vi "Connect to cDAQ.vi"(10 "System":string, 11 "Abort Ref":refnum<vi>) -> (1 "Abort":bool, 2 "Connected?":bool, 3 "System Ref":tag)   [LabVIEW 2023]
uses:
  <resource>/objmgr/daqmx.rc
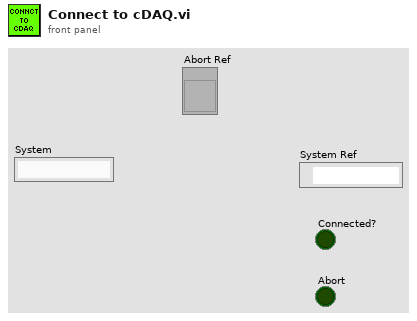
[diagram p1: front panel]
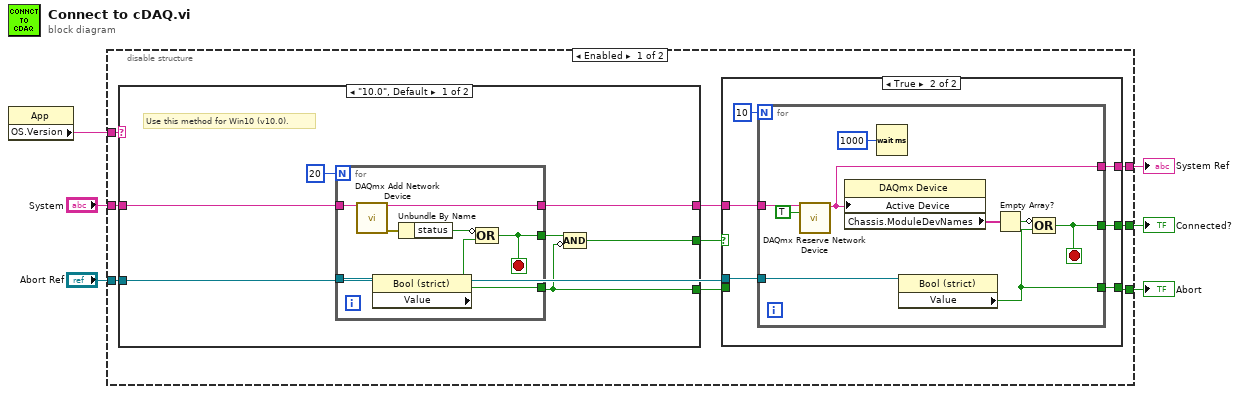
[diagram p0: block diagram]
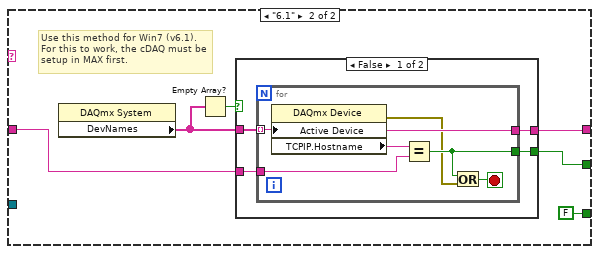
[diagram p2: hidden frame]
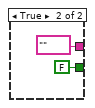
[diagram p3: hidden frame]
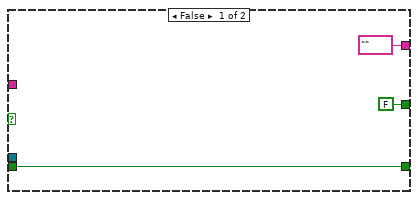
[diagram p4: hidden frame]
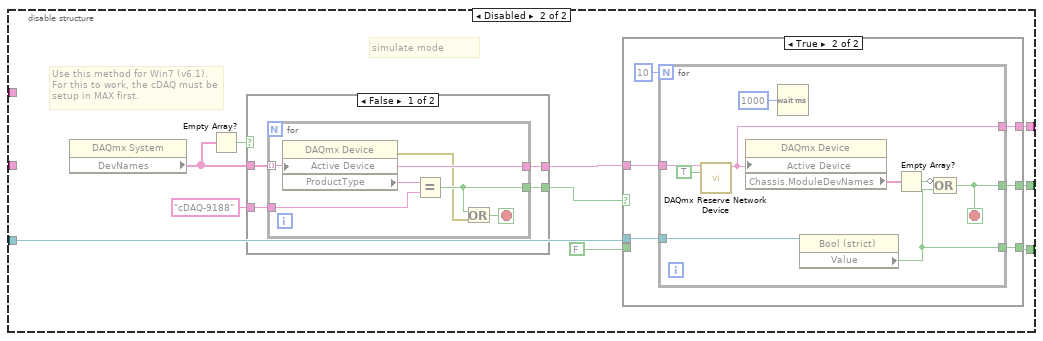
[diagram p5: hidden frame]
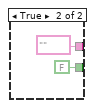
[diagram p6: hidden frame]
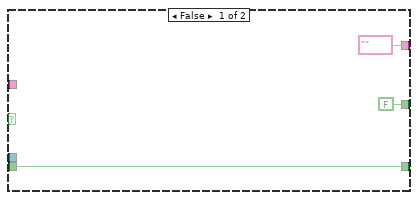
[diagram p7: hidden frame]
diagram:
  n1 = property class="App"() -> ("OS.Version"=w1:string)  [unwired: 2 in, 2 out]
  n2 = disable-structure shown="Enabled" {
    disable-tunnel: "System" -> [w15 _]
    disable-tunnel: [w12 w73] -> w5
    disable-tunnel: [w11 w72] -> w4
    disable-tunnel: [w10 w71] -> w3
    disable-tunnel: "Abort Ref" -> [w8 w69]
    disable-tunnel: w1 -> [w7 _]
    frame Enabled {
      n3 = case shown="\"10.0\", Default" w7 {
        tunnel: w15 -> [w22 w30]
        tunnel: [w21 FALSE ("Value")] -> w14
        tunnel: [w20 w32] -> w13
        tunnel: [w19 w33] -> w9
        tunnel: w8 -> [w18 _]
        frame "10.0", Default {
          # "Use this method for Win10 (v10.0)."
          n4 = for {
            N: 20 -> [_]
            tunnel: [w26] -> w16
            tunnel: [w28] -> w19
            tunnel: w22 -> [w24]
            tunnel: [w25] -> w21
            tunnel: w18 -> [w23]
            stop <- w26 stop-if-true
            n5 = call <vilib>:"DAQmx Add Network Device.vi"("device IP address/hostname"=w24) -> ("device out"=w28:tag, "error out"=w29:errorcluster)  [unwired: 13 in]
            n6 = property class="Bool (strict)"(reference=w23) -> ("Value"=w25:bool)  [unwired: 1 in, 2 out]
            n7 = Unbundle By Name(w29) -> ("status"=w27:bool)
            n8 = Compound Arithmetic op=OR(invert w27, w25) -> (w26:bool)
          }
          n9 = Compound Arithmetic op=AND(w16, invert w21) -> (w20:bool)
        }
        frame "6.1" {
          # "Use this method for Win7 (v6.1).\nFor this to work, the cDAQ must be\nsetup in MAX first."
          n10 = property class="DAQmx System"() -> ("DevNames"=w35:tag[])  [unwired: 2 in, 2 out]
          n11 = Empty Array?(array=w35) -> (empty?=w34:bool)
          n12 = case shown="False" w34 {
            tunnel: w35 -> [w39 _]
            tunnel: w30 -> [w38 _]
            tunnel: [w37 FALSE] -> w32
            tunnel: [w36 tag ""] -> w33
            frame False {
              n13 = for {
                tunnel: w39 -> [w43] mode=indexing
                tunnel: w38 -> [w44]
                tunnel: [w42] -> w37
                tunnel: [w43] -> w36
                stop <- w40 stop-if-true
                n14 = property class="DAQmx Device"("Active Device"=w43) -> (error out=w41:errorcluster, "TCPIP.Hostname"=w45:string)  [unwired: 2 in, 1 out]
                n15 = Equal?(x=w45, y=w44) -> (x = y?=w42:bool)
                n16 = Or(x=w42, y=w41) -> (x .or. y?=w40:bool)
              }
            }
            frame True {
            }
          }
        }
      }
      n17 = case shown="True" w13 {
        tunnel: w9 -> [_ w56]
        tunnel: [FALSE w54] -> w10
        tunnel: [tag "" ("device out") w53] -> w11
        tunnel: w14 -> [w48 _]
        tunnel: [w48 w52] -> w12
        tunnel: w8 -> [_ w51]
        frame False {
        }
        frame True {
          n18 = for {
            N: 10 -> [_]
            tunnel: w56 -> [w64]
            tunnel: [w59] -> w54
            tunnel: [w61] -> w53
            tunnel: [w58] -> w52
            tunnel: w51 -> [w57]
            stop <- w59 stop-if-true
            n19 = call <vilib>:"DAQmx Reserve Network Device.vi"("device in"=w64, "override reservation?"=TRUE) -> ("device out"=w61:tag)  [unwired: 12 in, 1 out]
            n20 = property class="DAQmx Device"("Active Device"=w61) -> ("Chassis.ModuleDevNames"=w63:tag[])  [unwired: 2 in, 2 out]
            n21 = Wait (ms)(milliseconds to wait=u32 1000) -> ()  [unwired: 1 out]
            n22 = property class="Bool (strict)"(reference=w57) -> ("Value"=w58:bool)  [unwired: 1 in, 2 out]
            n23 = Empty Array?(array=w63) -> (empty?=w60:bool)
            n24 = Compound Arithmetic op=OR(invert w60, w58) -> (w59:bool)
          }
        }
      }
    }
    frame Disabled {
      # "simulate mode"
      # "Use this method for Win7 (v6.1).\nFor this to work, the cDAQ must be\nsetup in MAX first."
      n25 = property class="DAQmx System"() -> ("DevNames"=w68:tag[])  [unwired: 2 in, 2 out]
      n26 = Empty Array?(array=w68) -> (empty?=w67:bool)
      n27 = case shown="False" w67 {
        tunnel: w68 -> [w79 _]
        tunnel: "cDAQ-9188" ("System") -> [w78 _]
        tunnel: [w77 FALSE] -> w74
        tunnel: [w76 tag ""] -> w70
        frame False {
          n28 = for {
            tunnel: w79 -> [w83] mode=indexing
            tunnel: w78 -> [w84]
            tunnel: [w82] -> w77
            tunnel: [w83] -> w76
            stop <- w80 stop-if-true
            n29 = property class="DAQmx Device"("Active Device"=w83) -> (error out=w81:errorcluster, "ProductType"=w85:string)  [unwired: 2 in, 1 out]
            n30 = Equal?(x=w85, y=w84) -> (x = y?=w82:bool)
            n31 = Or(x=w82, y=w81) -> (x .or. y?=w80:bool)
          }
        }
        frame True {
        }
      }
      n32 = case shown="True" w74 {
        tunnel: w70 -> [_ w96]
        tunnel: [FALSE w94] -> w71
        tunnel: [tag "" ("device out") w93] -> w72
        tunnel: FALSE ("Value") -> [w88 _]
        tunnel: [w88 w92] -> w73
        tunnel: w69 -> [_ w91]
        frame False {
        }
        frame True {
          n33 = for {
            N: 10 -> [_]
            tunnel: w96 -> [w104]
            tunnel: [w99] -> w94
            tunnel: [w101] -> w93
            tunnel: [w98] -> w92
            tunnel: w91 -> [w97]
            stop <- w99 stop-if-true
            n34 = call <vilib>:"DAQmx Reserve Network Device.vi"("device in"=w104, "override reservation?"=TRUE) -> ("device out"=w101:tag)  [unwired: 12 in, 1 out]
            n35 = property class="DAQmx Device"("Active Device"=w101) -> ("Chassis.ModuleDevNames"=w103:tag[])  [unwired: 2 in, 2 out]
            n36 = Wait (ms)(milliseconds to wait=u32 1000) -> ()  [unwired: 1 out]
            n37 = property class="Bool (strict)"(reference=w97) -> ("Value"=w98:bool)  [unwired: 1 in, 2 out]
            n38 = Empty Array?(array=w103) -> (empty?=w100:bool)
            n39 = Compound Arithmetic op=OR(invert w100, w98) -> (w99:bool)
          }
        }
      }
    }
  }
  "Abort" <- w5
  "System Ref" <- w4
  "Connected?" <- w3
